vi "数据处理.vi"(11 "数据输入":string[](array[string])) -> (3 "数据输出":string[](array[string]))   [LabVIEW 2011]
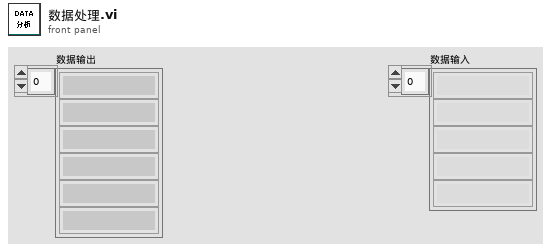
[diagram p1: front panel]
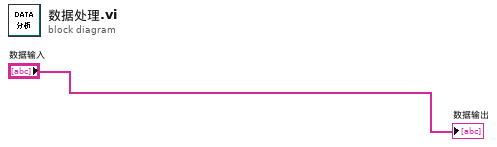
[diagram p0: block diagram]
diagram:
  "数据输出" <- "数据输入"
